vi "ratelimiter.vi"(8 "Ts":dbl=0.005, 9 "falling slew rate":dbl, 10 "rising slew rate":dbl, 11 "input":dbl) -> (0 "input(k-1)":dbl, 3 "output":dbl)   [LabVIEW 2012]
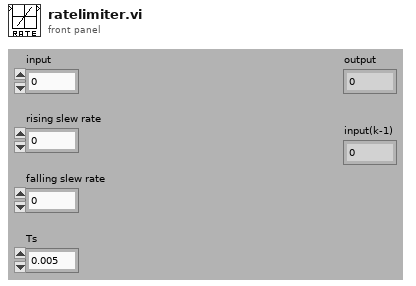
[diagram p1: front panel]
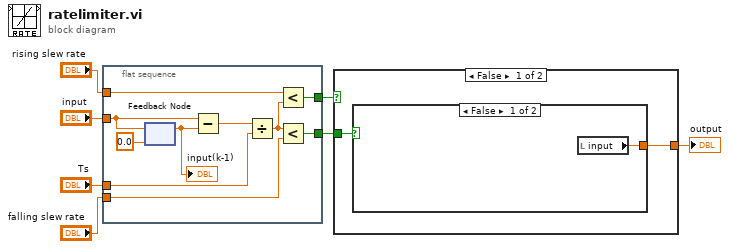
[diagram p0: block diagram]
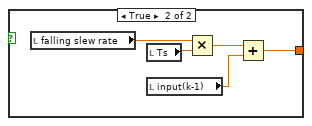
[diagram p2: hidden frame]
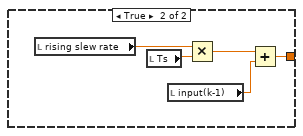
[diagram p3: hidden frame]
diagram:
  n1 = flat-sequence {
    tunnel: "input" -> [w16]
    tunnel: "rising slew rate" -> [w13]
    tunnel: [w12] -> w5
    tunnel: "Ts" -> [w11]
    tunnel: "falling slew rate" -> [w10]
    tunnel: [w8] -> w2
    frame #0 {
      n2 = feedback #1(0.0 ("input")) -> (w15:dbl)
      "input(k-1)" <- w15
      n3 = feedback-in #1(w16) -> ()
      n4 = Subtract(x=w16, y=w15) -> (x-y=w14:dbl)
      n5 = Divide(x=w14, y=w11) -> (x/y=w9:dbl)
      n6 = Less?(x=w13, y=w9) -> (x < y?=w12:bool)
      n7 = Less?(x=w9, y=w10) -> (x < y?=w8:bool)
    }
  }
  n8 = case shown="False" w5 {
    tunnel: w2 -> [w19 _]
    tunnel: [w18 w26] -> w1
    frame False {
      n9 = case shown="False" w19 {
        tunnel: [w20 w21] -> w18
        frame False {
          n10 = local read "input"() -> (w20:dbl)
        }
        frame True {
          n11 = local read "falling slew rate"() -> (w25:dbl)
          n12 = local read "Ts"() -> (w24:dbl)
          n13 = local read "input(k-1)"() -> (w22:dbl)
          n14 = Multiply(x=w25, y=w24) -> (x*y=w23:dbl)
          n15 = Add(x=w23, y=w22) -> (x+y=w21:dbl)
        }
      }
    }
    frame True {
      n16 = local read "rising slew rate"() -> (w30:dbl)
      n17 = local read "Ts"() -> (w29:dbl)
      n18 = local read "input(k-1)"() -> (w27:dbl)
      n19 = Multiply(x=w30, y=w29) -> (x*y=w28:dbl)
      n20 = Add(x=w28, y=w27) -> (x+y=w26:dbl)
    }
  }
  "output" <- w1
